vi "jenkins_unit_test.vi"(11 "Args":string[](array[string])) -> (2 "Output":string, 3 "Exit Code":i32)   [LabVIEW 2019]
uses:
  <vilib>/addons/_JKI Toolkits/Caraya/classes/Test Suite/Define Test Suite (JUnit Report).vi
  <vilib>/addons/_JKI Toolkits/Caraya/classes/Test Suite/Test Suite.lvclass
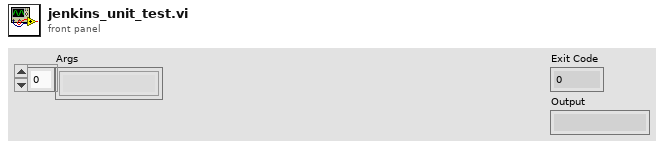
[diagram p1: front panel]
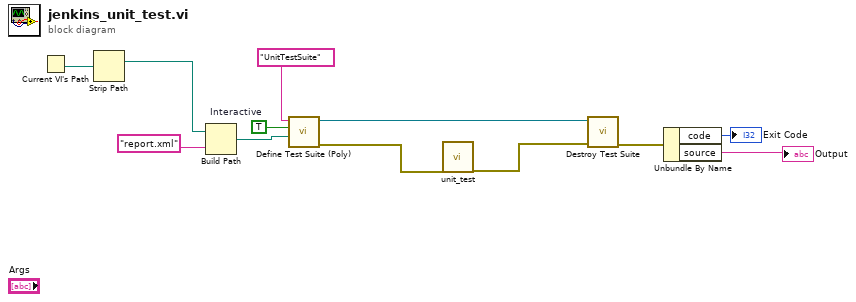
[diagram p0: block diagram]
diagram:
  w10 = TRUE  # Interactive
  n1 = Current VI's Path() -> (path=w3:path)
  n2 = Strip Path(path=w3) -> (stripped path=w1:path)  [unwired: 1 out]
  n3 = Build Path(base path=w1, name or relative path="report.xml") -> (appended path=w11:path)
  n4 = call-poly <vilib>:"Define Test Suite (Poly).vi"("Report Path"=w11, "Interactive"=w10, "Label (VI Title)"="UnitTestSuite") -> ("error out"=w8:errorcluster, "Test Suite"=w9:refnum<class "Test Suite.lvclass">)  [unwired: 7 in]
  n5 = call "unit_test.vi"("error in (no error)"=w8) -> ("error out"=w7:errorcluster)  [unwired: 10 in]
  n6 = call-dynamic "Destroy Test Suite.vi"("error in (no error)"=w7, "Test Suite in"=w9) -> ("error out"=w6:errorcluster)  [unwired: 8 in, 1 out]
  n7 = Unbundle By Name(w6) -> ("code"=→"Exit Code":i32, "source"=→"Output":string)
